vi "example_init.vi"(0 "Spectroscopy Cluster":T2={"Mode"=0, "Start [a.u.]"=-inf, "End [a.u.]"=-inf, "Points"=-2147483648, "Repeat"=-2147483648, "Fwd/Bwd"=FALSE, "Delay"=-inf, "Preferences Button"=FALSE, "DAC"=0, "Avg Time"=-inf} {"Avg Time" format="%#_g µs"; "DAC" items=["DAC 1"=0, "DAC 2"=1, "DAC 3"=2, "DAC 4"=3, "Z"=26, "Low Frequency"=27]; "Delay" format="%#_g µs"; "Mode" items=["Spectroscopy 1", "Spectroscopy 2", "Spectroscopy 3", "Calibration"]}, 5 "Source for permanent":T1 items=["[read only]"=-2147483648, "ADC 1"=0, "ADC 2"=1, "ADC 3"=2, "ADC 4"=3, "ADC 5"=4, "ADC 6"=5, "HF 1 Out"=7, "HF 1 df"=8, "z out"=9, "HF 1"=12, "HF 1 Ampl."=13, "HF 1 Phase"=14, "LF LockIn Ampl"=16, "LF LockIn Phase"=17, "z out inv"=18, "counter"=23, "Crosslink 1"=29, "Crosslink 2"=30, "Pos X"=31, "Pos Y"=32], 11 "error in":T6) -> (2 "Scan Cluster":T5={"Lines"=-2147483648, "Columns"=-2147483648, "X Range "=-inf, "Y Range "=-inf, "Pixel Size"=-inf, "Origin X"=-inf, "Origin Y"=-inf, "Rotation"=-inf, "Sample Time"=-inf} {"Sample Time" format="%#_g µs"; "Rotation" format="%#_g deg"; "Origin Y" format="%#_g nm"; "Origin X" format="%#_g nm"; "Pixel Size" format="%#_g nm"; "Y Range" format="%#_g nm"; "X Range" format="%#_g nm"; "Columns" max=250; "Lines" max=250}, 3 "Spectroscopy Cluster":T2={"Mode"=0, "Start [a.u.]"=-inf, "End [a.u.]"=-inf, "Points"=-2147483648, "Repeat"=-2147483648, "Fwd/Bwd"=FALSE, "Delay"=-inf, "Preferences Button"=FALSE, "DAC"=0, "Avg Time"=-inf} {"Avg Time" format="%#_g µs"; "DAC" items=["DAC 1"=0, "DAC 2"=1, "DAC 3"=2, "DAC 4"=3, "Z"=26, "Low Frequency"=27]; "Delay" format="%#_g µs"; "Mode" items=["Spectroscopy 1", "Spectroscopy 2", "Spectroscopy 3", "Calibration"]}, 4 "temperature":sgl, 6 "Output Status":bool, 8 "CorrespondingChScan":i32[](array[numeric])=[0, 1], 10 "SourceText_ChNumScan":cluster{"RingText.Text":string, i32}[](array[cluster])=[{"RingText.Text"="ADC 2", 0}, {"RingText.Text"="ADC 1", 1}], 13 "CorrespondingChSpec":i32[](array[numeric]), 14 "SourceText_ChNumSpec":cluster{"RingText.Text":string, i32}[](array[cluster])=[{"RingText.Text"="ADC 2", 0}, {"RingText.Text"="ADC 1", 1}], 15 "error out":T6)   [LabVIEW 2016]
uses:
  Controls/Error_Out.ctl
  Controls/Spectroscopy_Parameters.ctl
  Controls/Spectroscopy-Mode_Selection.ctl
  Controls/Spec_DAC_Selection.ctl
  Controls/Scan_Parameters.ctl
  Controls/Channel-Source_Selection.ctl
  Controls/Channel_Parameters.ctl
  Controls/Channel_Selection.ctl
  Controls/Average_Selection.ctl
  Controls/Trigger_Selection.ctl
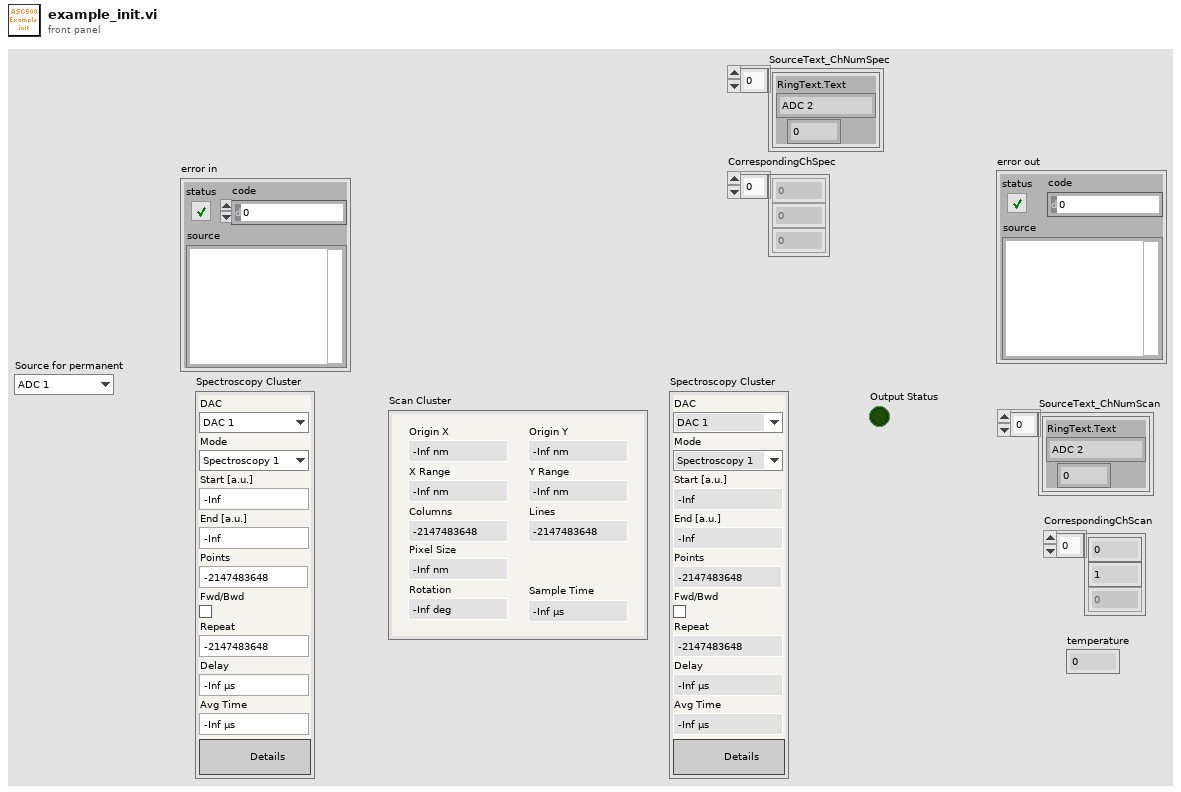
[diagram p1: front panel]
types:
  T1 = typedef "Channel-Source_Selection.ctl" = i32
  T2 = typedef "Spectroscopy_Parameters.ctl" = cluster{"Mode":T3, "Start [a.u.]":sgl, "End [a.u.]":sgl, "Points":i32, "Repeat":i32, "Fwd/Bwd":bool, "Delay":sgl, "Preferences Button":bool, "DAC":T4, "Avg Time":sgl}
  T3 = typedef "Spectroscopy-Mode_Selection.ctl" = u16
  T4 = typedef "Spec_DAC_Selection.ctl" = u16
  T5 = typedef "Scan_Parameters.ctl" = cluster{"Lines":i32, "Columns":i32, "X Range ":sgl, "Y Range ":sgl, "Pixel Size":sgl, "Origin X":sgl, "Origin Y":sgl, "Rotation":sgl, "Sample Time":sgl}
  T6 = typedef "Error_Out.ctl" = errorcluster
  T7 = enum32{"Disabled", "Scan", "Line", "Spec 1", "Spec 2", "Spec 3", "Cal", "Trigger", "Every", "SoftSpec", "DualPass", "Step Scan"}
  T8 = typedef "Channel_Parameters.ctl" = cluster{"Channel":T9, "Source":T1, "Average":T10, "SampleTime [us]":sgl, "Trigger":T11}
  T9 = typedef "Channel_Selection.ctl" = i32
  T10 = typedef "Average_Selection.ctl" = i32
  T11 = typedef "Trigger_Selection.ctl" = i32
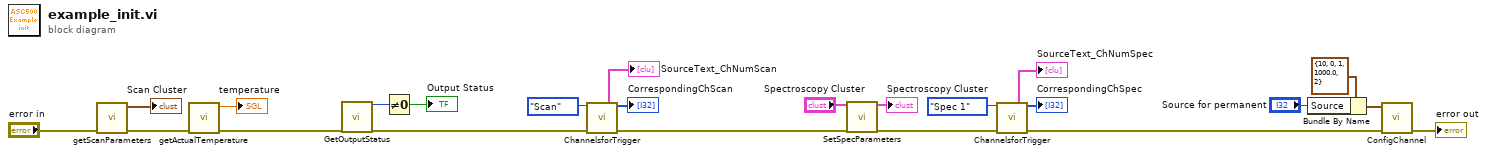
[diagram p0: block diagram]
diagram:
  n1 = call "getScanParameters.vi"("error in"="error in") -> ("error out"=w6:T6, "Output Scan Cluster"=→"Scan Cluster":T5)  [unwired: 9 in]
  n2 = call "getActualTemperature.vi"("error in"=w6) -> ("error out"=w4:T6, "temperature"=→"temperature":sgl)  [unwired: 9 in]
  n3 = call "GetOutputStatus.vi"("error in"=w4) -> ("Status out"=w2:i32, "error out"=w3:T6)  [unwired: 17 in]
  n4 = Not Equal To 0?(x=w2) -> (x != 0?=→"Output Status":bool)
  n5 = call "ChannelsforTrigger.vi"("Trigger"=T7."Scan", "error in"=w3) -> ("SourceText_ChNum"=→"SourceText_ChNumScan":cluster{"RingText.Text":string, i32}[], "Corresponding channels"=→"CorrespondingChScan":i32[], "error out"=w21:T6)  [unwired: 8 in, 3 out]
  n6 = call "SetSpecParameters.vi"("Spectroscopy Cluster"="Spectroscopy Cluster", "error in"=w21) -> ("Output Cluster"=→"Spectroscopy Cluster":T2, "error out"=w11:T6)  [unwired: 16 in]
  n7 = call "ChannelsforTrigger.vi"("Trigger"=T7."Spec 1", "error in"=w11) -> ("SourceText_ChNum"=→"SourceText_ChNumSpec":cluster{"RingText.Text":string, i32}[], "Corresponding channels"=→"CorrespondingChSpec":i32[], "error out"=w10:T6)  [unwired: 8 in, 3 out]
  n8 = Bundle By Name(cluster=T8 {"Channel"=10, "Source"=0, "Average"=1, "SampleTime [us]"=1000.0, "Trigger"=2} ("Channel Cluster"), "Source"="Source for permanent") -> (w15:T8)
  n9 = call "ConfigChannel.vi"("error in"=w10, "Channel Cluster"=w15) -> ("error out"=→"error out":T6)  [unwired: 8 in, 1 out]
